vi "ChannelNameStringToEnum.vi"(11 "ChannelName":string) -> (3 "Channel (0: Channel 1)":T1 items=["Channel 1", "Channel 2", "Channel 3", "Channel 4", "Math", "Reference 1", "Reference 2", "Reference 3", "Reference 4", "Bus 1", "Bus 2"])   [LabVIEW 2013, in "TektronixDPO.lvclass"]
uses:
  TektronixDPO.lvclass
  shared/Typdefs/Choice80.ctl
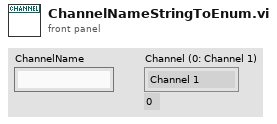
[diagram p1: front panel]
types:
  T1 = typedef "Choice80.ctl" = u16
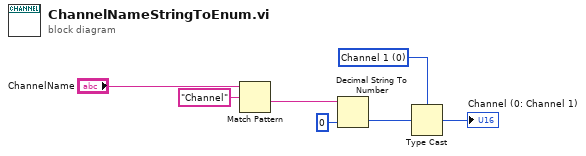
[diagram p0: block diagram]
diagram:
  w6 = T1 0 items=["Channel 1", "Channel 2", "Channel 3", "Channel 4", "Math", "Reference 1", "Reference 2", "Reference 3", "Reference 4", "Bus 1", "Bus 2"] ("Channel (0: Channel 1)")
  n1 = Match Pattern(string="ChannelName", regular expression="Channel") -> (after substring=w4:string)  [unwired: 1 in, 3 out]
  n2 = Decimal String To Number(string=w4, default (0L)=u16 0 ("default (0 I32)")) -> (number=w1:u16)  [unwired: 1 in, 1 out]
  n3 = Type Cast(type=w6, x=w1) -> (*(type *) &x=→"Channel (0: Channel 1)":T1)
